vi "QBridge 0MQ focuser.vi"() -> (0 "error":errorcluster)   [LabVIEW 2018]
uses:
  <vilib>/addons/zeromq/zmq_socket.lvclass
  <vilib>/addons/zeromq/zmq_context.lvclass
  <vilib>/addons/zeromq/socket_type.ctl
  <vilib>/addons/zeromq/socket_options.ctl
  <vilib>/addons/zeromq/zeromq.lvlib
panel:
  out "focuserREP message":string
  out "Focuser160_REQ":string caption="Message to Focuser160"
  out "Focus Status":string
  in  "QueueBaseName":string="focusQueue"
  in  "stop":bool
  # "QBRIDGE ZeroMQ Focuser"
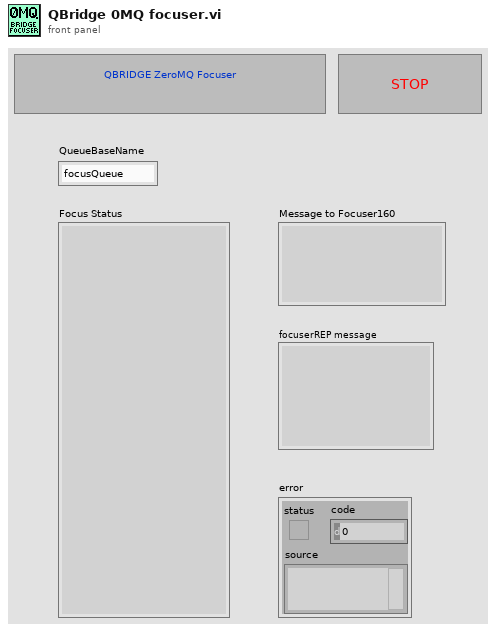
[diagram p1: front panel]
types:
  T1 = typedef "zeromq.lvlib/socket_options.ctl" = enum8{"NONE", "ZMQ_HWM", "<2>", "ZMQ_SWAP", "ZMQ_AFFINITY", "ZMQ_ROUTING_ID", "ZMQ_SUBSCRIBE", "ZMQ_UNSUBSCRIBE", "ZMQ_RATE", "ZMQ_RECOVERY_IVL", "ZMQ_MCAST_LOOP", "ZMQ_SNDBUF", "ZMQ_RCVBUF", "ZMQ_RCVMORE", "ZMQ_FD", "ZMQ_EVENTS", "ZMQ_TYPE", "ZMQ_LINGER", "ZMQ_RECONNECT_IVL", "ZMQ_BACKLOG", "ZMQ_RECOVERY_IVL_MSEC", "ZMQ_RECONNECT_IVL_MAX", "ZMQ_MAXMSGSIZE", "ZMQ_SNDHWM", "ZMQ_RCVHWM", "ZMQ_MULTICAST_HOPS", "<26>", "ZMQ_RCVTIMEO", "ZMQ_SNDTIMEO", "<29>", "<30>", "ZMQ_IPV4ONLY", "ZMQ_LAST_ENDPOINT", "ZMQ_ROUTER_MANDATORY", "ZMQ_TCP_KEEPALIVE", "ZMQ_TCP_KEEPALIVE_CNT", "ZMQ_TCP_KEEPALIVE_IDLE", "ZMQ_TCP_KEEPALIVE_INTVL", "ZMQ_TCP_ACCEPT_FILTER", "ZMQ_IMMEDIATE", "ZMQ_XPUB_VERBOSE", "ZMQ_ROUTER_RAW", "ZMQ_IPV6", "ZMQ_MECHANISM", "ZMQ_PLAIN_SERVER", "ZMQ_PLAIN_USERNAME", "ZMQ_PLAIN_PASSWORD", "ZMQ_CURVE_SERVER", "ZMQ_CURVE_PUBLICKEY", "ZMQ_CURVE_SECRETKEY", "ZMQ_CURVE_SERVERKEY", "ZMQ_PROBE_ROUTER", "ZMQ_REQ_CORRELATE", "ZMQ_REQ_RELAXED", "ZMQ_CONFLATE", "ZMQ_ZAP_DOMAIN", "ZMQ_ROUTER_HANDOVER", "ZMQ_TOS", "ZMQ_IPC_FILTER_PID", "ZMQ_IPC_FILTER_UID", "ZMQ_IPC_FILTER_GID", "ZMQ_CONNECT_ROUTING_ID", "ZMQ_GSSAPI_SERVER", "ZMQ_GSSAPI_PRINCIPAL", "ZMQ_GSSAPI_SERVICE_PRINCIPAL", "ZMQ_GSSAPI_PLAINTEXT", "ZMQ_HANDSHAKE_IVL", "<67>", "ZMQ_SOCKS_PROXY", "ZMQ_XPUB_NODROP", "ZMQ_BLOCKY", "ZMQ_XPUB_MANUAL", "ZMQ_XPUB_WELCOME_MSG", "ZMQ_STREAM_NOTIFY", "ZMQ_INVERT_MATCHING", "ZMQ_HEARTBEAT_IVL", "ZMQ_HEARTBEAT_TTL", "ZMQ_HEARTBEAT_TIMEOUT", "ZMQ_XPUB_VERBOSER", "ZMQ_CONNECT_TIMEOUT", "ZMQ_TCP_MAXRT", "ZMQ_THREAD_SAFE", "<82>", "<83>", "ZMQ_MULTICAST_MAXTPDU", "ZMQ_VMCI_BUFFER_SIZE", "ZMQ_VMCI_BUFFER_MIN_SIZE", "ZMQ_VMCI_BUFFER_MAX_SIZE", "ZMQ_VMCI_CONNECT_TIMEOUT", "ZMQ_USE_FD", "ZMQ_GSSAPI_PRINCIPAL_NAMETYPE", "ZMQ_GSSAPI_SERVICE_PRINCIPAL_NAMETYPE", "ZMQ_BINDTODEVICE", "ZMQ_ZAP_ENFORCE_DOMAIN", "ZMQ_LOOPBACK_FASTPATH", "ZMQ_METADATA", "ZMQ_MULTICAST_LOOP", "ZMQ_ROUTER_NOTIFY"}
  T2 = typedef "zeromq.lvlib/socket_type.ctl" = enum8{"ZMQ_PAIR", "ZMQ_PUB", "ZMQ_SUB", "ZMQ_REQ", "ZMQ_REP", "ZMQ_DEALER", "ZMQ_ROUTER", "ZMQ_PULL", "ZMQ_PUSH", "ZMQ_XPUB", "ZMQ_XSUB", "ZMQ_STREAM", "ZMQ_SERVER", "ZMQ_CLIENT", "ZMQ_RADIO", "ZMQ_DISH", "ZMQ_GATHER", "ZMQ_SCATTER", "ZMQ_DGRAM"}
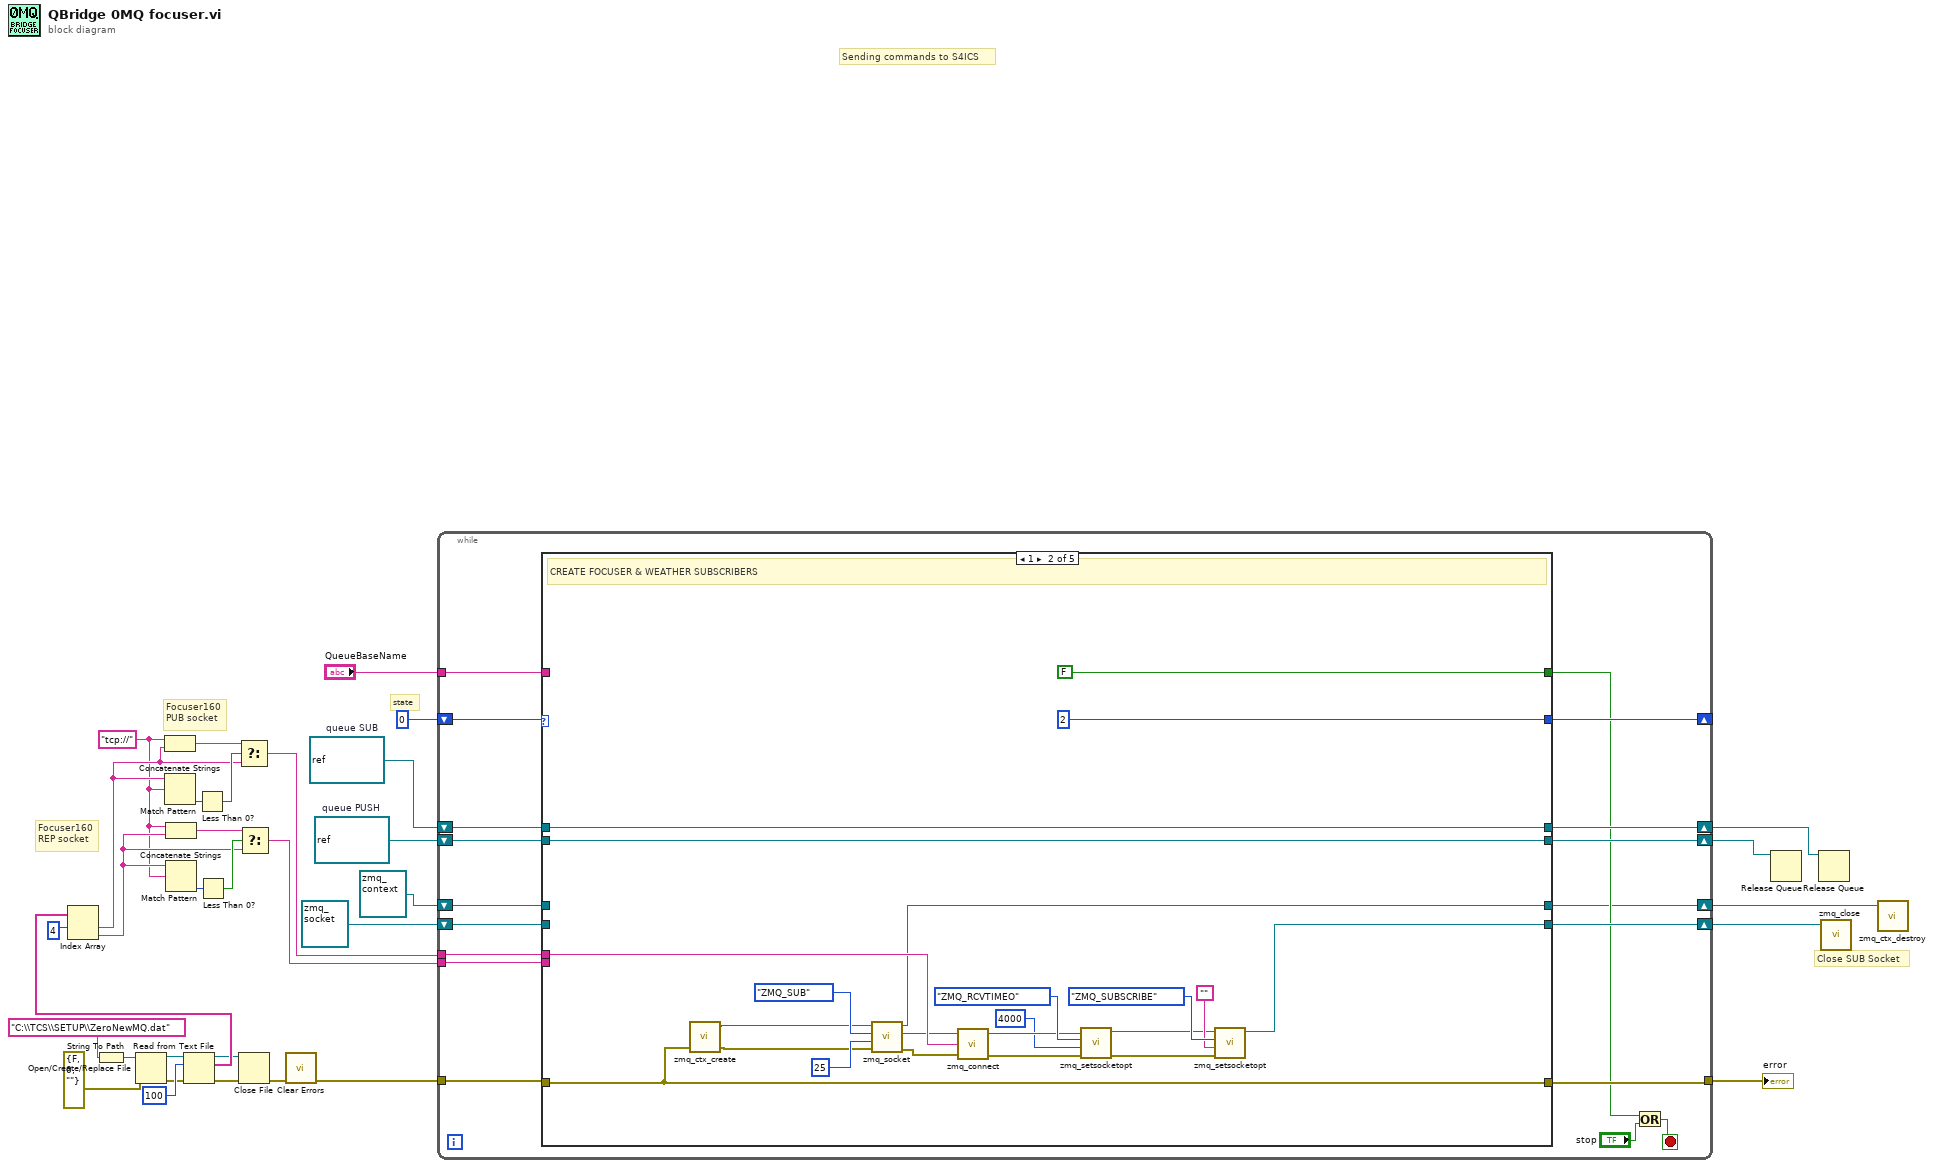
[diagram p0: block diagram]
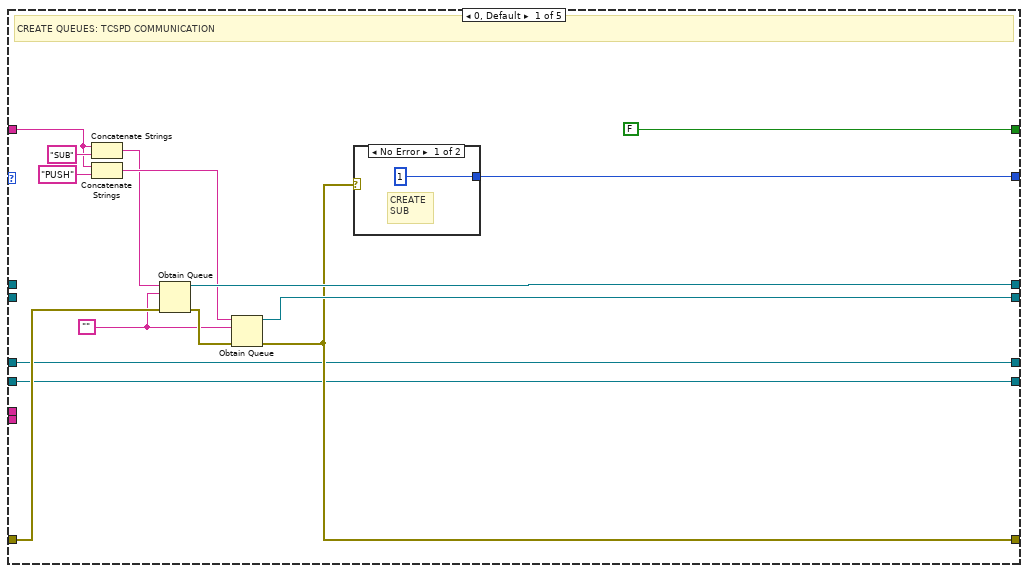
[diagram p2: hidden frame]
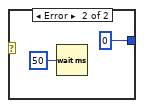
[diagram p3: hidden frame]
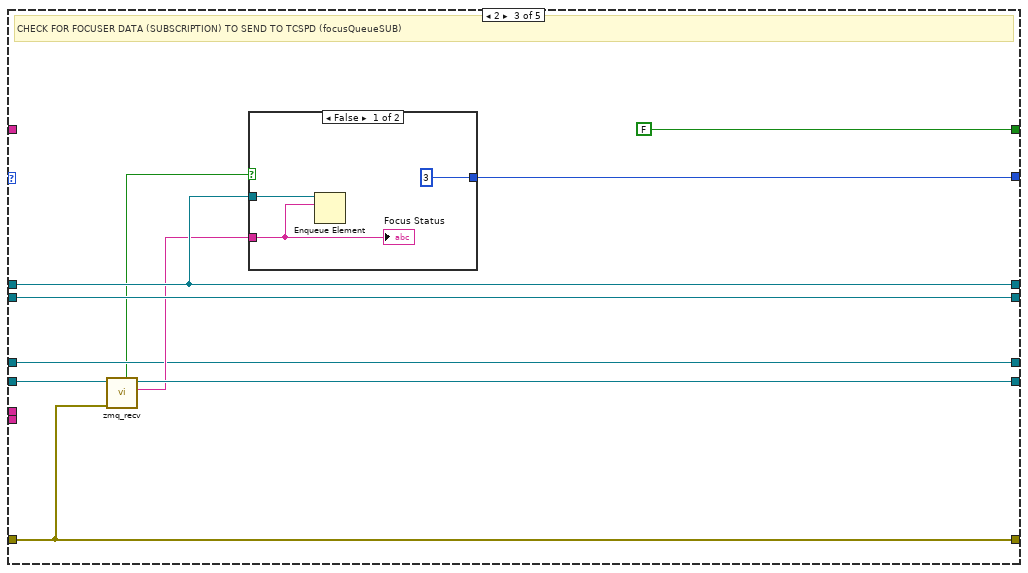
[diagram p4: hidden frame]
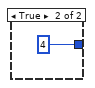
[diagram p5: hidden frame]
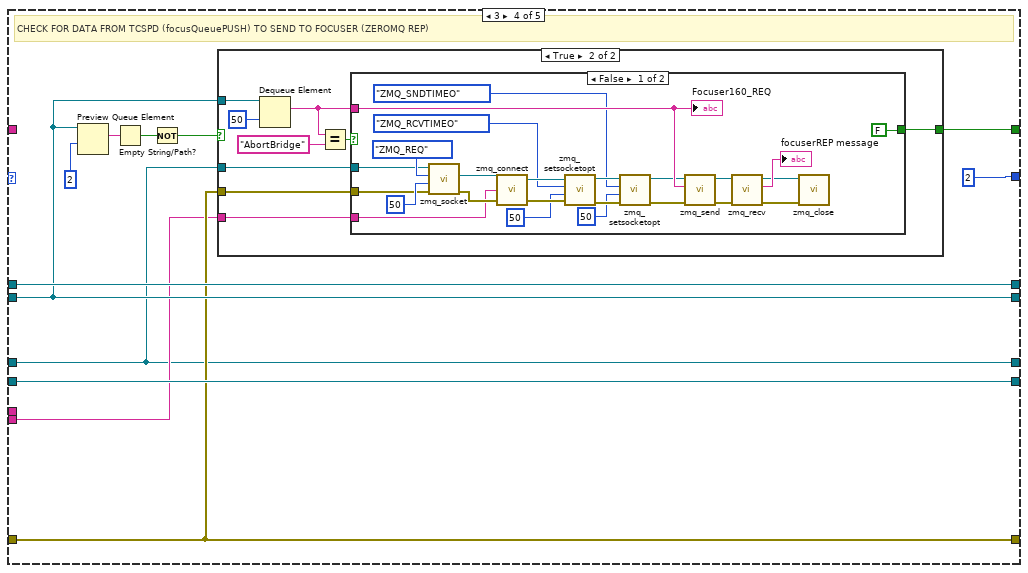
[diagram p6: hidden frame]
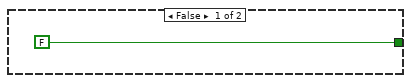
[diagram p7: hidden frame]
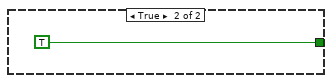
[diagram p8: hidden frame]
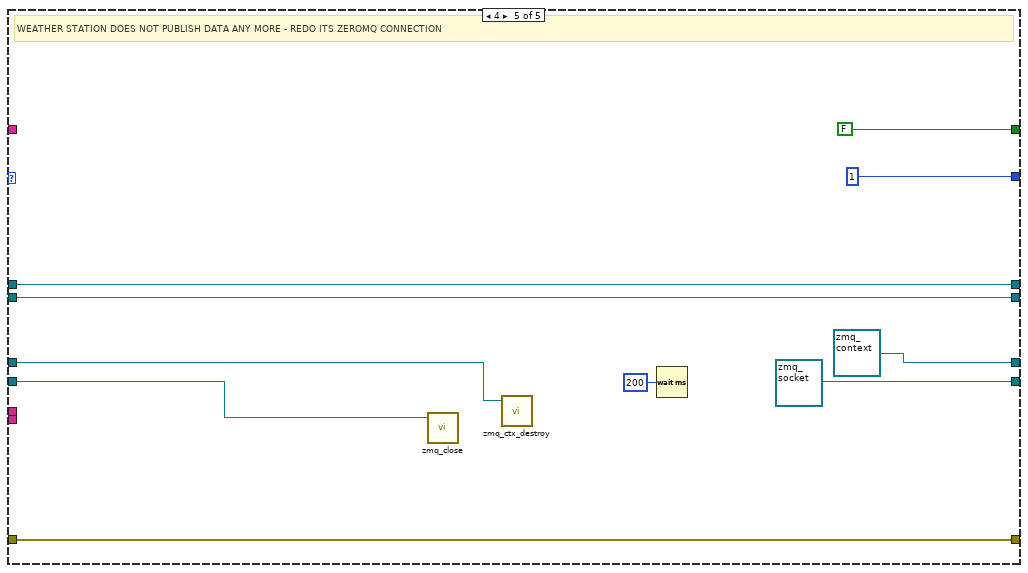
[diagram p9: hidden frame]
diagram:
  w4 = "tcp://"
  w32 = refnum<queue> refnum  # queue PUSH
  w31 = refnum<queue> refnum  # queue SUB
  # "Close SUB Socket"
  # "Focuser160\nREP socket"
  # "Focuser160\nPUB socket"
  # "state"
  # "Sending commands to S4ICS"
  n1 = String To Path(string="C:\\TCS\\SETUP\\ZeroNewMQ.dat") -> (path=w29:path)
  n2 = Open/Create/Replace File(file path (use dialog)=w29, error in=errorcluster {"status"=FALSE, "code"=0, "source"=""}) -> (refnum out=w27:refnum<file>, error out=w20:errorcluster)  [unwired: 4 in, 1 out]
  n3 = Read from Text File(file (use dialog)=w27, count=100, error in=w20) -> (refnum out=w23:refnum<file>, text=w25:string[], error out=w16:errorcluster)  [unwired: 1 in, 1 out]
  n4 = Index Array(array=w25, index #1=4 ("index")) -> (element #1=w6:string, element #2=w11:string)  [unwired: 1 in]
  n5 = Concatenate Strings(w4, w6) -> (w8:string)
  n6 = Match Pattern(string=w6, regular expression=w4) -> (offset past match=w7:i32)  [unwired: 1 in, 3 out]
  n7 = Concatenate Strings(w4, w11) -> (w13:string)
  n8 = Match Pattern(string=w11, regular expression=w4) -> (offset past match=w12:i32)  [unwired: 1 in, 3 out]
  n9 = Less Than 0?(x=w7) -> (x < 0?=w9:bool)
  n10 = Less Than 0?(x=w12) -> (x < 0?=w14:bool)
  n11 = Select(t=w8, s=w9, f=w6) -> (s? t:f=w5:string)
  n12 = Close File(refnum=w23, error in=w16) -> (error out=w17:errorcluster)  [unwired: 1 out]
  n13 = Select(t=w13, s=w14, f=w11) -> (s? t:f=w10:string)
  n14 = call <vilib>:"Clear Errors.vi"("error in (no error)"=w17) -> ("error out"=w3:errorcluster)  [unwired: 5 in, 1 out]
  n15 = while {
    shift-right: [w50] -> _
    shift-left: u16 0 -> [w52]
    shift-right: [w46] -> w19
    shift-left: w31 -> [w44]
    shift-right: [w45] -> w18
    shift-left: w32 -> [w43]
    tunnel: w3 -> [w51]
    tunnel: [w49] -> w33
    tunnel: "QueueBaseName" -> [w42]
    tunnel: w5 -> [w41]
    tunnel: w10 -> [w40]
    shift-right: [w38] -> w15
    shift-left: refnum<class "zmq_socket.lvclass"> refnum ("socket out") -> [w39]
    shift-right: [w35] -> w1
    shift-left: refnum<class "zmq_context.lvclass"> refnum ("context out") -> [w36]
    stop <- w47 stop-if-true
    n16 = case shown="1" w52 {
      tunnel: w51 -> [w64 w81 w97 w112 w161]
      tunnel: [w65 u16 2 w93 u16 2 u16 1] -> w50
      tunnel: [w62 w81 w97 w112 w161] -> w49
      tunnel: [w67 w91 w99 w118 w163] -> w46
      tunnel: [w66 w90 w102 w114 w162] -> w45
      tunnel: w44 -> [_ w91 w99 w118 w163]
      tunnel: w43 -> [_ w90 w102 w114 w162]
      tunnel: w42 -> [w56 _ _ _ _]
      tunnel: w41 -> [_ w88 _ _ _]
      tunnel: w40 -> [_ _ _ w109 _]
      tunnel: w39 -> [w55 _ w101 w113 w158]
      tunnel: [w55 w92 w100 w113 refnum<class "zmq_socket.lvclass"> refnum ("socket out")] -> w38
      tunnel: [FALSE FALSE FALSE w111 FALSE] -> w37
      tunnel: w36 -> [w53 _ w95 w107 w157]
      tunnel: [w53 w77 w95 w107 refnum<class "zmq_context.lvclass"> refnum ("context out")] -> w35
      frame 0, Default {
        w57 = ""
        # "CREATE QUEUES: TCSPD COMMUNICATION"
        n17 = Concatenate Strings(w56, "SUB" ("string")) -> (w58:string)
        n18 = Concatenate Strings(w56, "PUSH" ("string")) -> (w60:string)
        n19 = Obtain Queue(name (unnamed)=w58, element data type=w57, error in (no error)=w64) -> (queue out=w67:refnum<queue>, error out=w63:errorcluster)  [unwired: 2 in, 1 out]
        n20 = Obtain Queue(name (unnamed)=w60, element data type=w57, error in (no error)=w63) -> (queue out=w66:refnum<queue>, error out=w62:errorcluster)  [unwired: 2 in, 1 out]
        n21 = case shown="No Error" w62 {
          tunnel: [u16 1 u16 0] -> w65
          frame No Error {
            # "CREATE\nSUB"
          }
          frame Error {
            n22 = Wait (ms)(milliseconds to wait=u32 50) -> ()  [unwired: 1 out]
          }
        }
      }
      frame 1 {
        # "CREATE FOCUSER & WEATHER SUBSCRIBERS"
        n23 = call <vilib>:"zmq_ctx_create.vi"("error in"=w81) -> ("error out"=w78:errorcluster, "context out"=w79:refnum<class "zmq_context.lvclass">)  [unwired: 3 in]
        n24 = call <vilib>:"zmq_socket.vi"("error in"=w78, "linger (ms)"=25, "socket type"=socket_type."ZMQ_SUB", "context in"=w79) -> ("error out"=w86:errorcluster, "socket out"=w87:refnum<class "zmq_socket.lvclass">, "context out"=w77:refnum<class "zmq_context.lvclass">)  [unwired: 1 in]
        n25 = call <vilib>:"zmq_connect.vi"("error in"=w86, "endpoint"=w88, "socket in"=w87) -> ("error out"=w72:errorcluster, "socket out"=w75:refnum<class "zmq_socket.lvclass">)  [unwired: 1 in]
        n26 = call <vilib>:"zmq_setsocketopt.vi"("error in"=w72, "value"=u16 4000, "option"=socket_options."ZMQ_RCVTIMEO", "socket in"=w75) -> ("error out"=w73:errorcluster, "socket out"=w74:refnum<class "zmq_socket.lvclass">)  [unwired: 2 in]
        n27 = call <vilib>:"zmq_setsocketopt.vi"("error in"=w73, "value"="", "option"=socket_options."ZMQ_SUBSCRIBE", "socket in"=w74) -> ("socket out"=w92:refnum<class "zmq_socket.lvclass">)  [unwired: 2 in, 1 out]
      }
      frame 2 {
        # "CHECK FOR FOCUSER DATA (SUBSCRIPTION) TO SEND TO TCSPD (focusQueueSUB)"
        n28 = call <vilib>:"zmq_recv.vi"("error in"=w97, "socket in"=w101) -> ("data"=w96:string, "socket out"=w100:refnum<class "zmq_socket.lvclass">, "timeout?"=w94:bool)  [unwired: 3 in, 2 out]
        n29 = case shown="False" w94 {
          tunnel: w99 -> [w105 _]
          tunnel: w96 -> [w104 _]
          tunnel: [u16 3 u16 4] -> w93
          frame False {
            n30 = Enqueue Element(queue=w105, element=w104) -> ()  [unwired: 2 in, 3 out]
            "Focus Status" <- w104
          }
          frame True {
          }
        }
      }
      frame 3 {
        # "CHECK FOR DATA FROM TCSPD (focusQueuePUSH) TO SEND TO FOCUSER (ZEROMQ REP)"
        n31 = Preview Queue Element(queue=w114, timeout in ms (-1)=2) -> (element=w117:string)  [unwired: 1 in, 3 out]
        n32 = Empty String/Path?(string/path=w117) -> (empty?=w116:bool)
        n33 = Not(x=w116) -> (.not. x?=w115:bool)
        n34 = case shown="True" w115 {
          tunnel: w114 -> [_ w128]
          tunnel: w109 -> [_ w126]
          tunnel: w112 -> [_ w127]
          tunnel: [FALSE w122] -> w111
          tunnel: w107 -> [_ w120]
          frame False {
          }
          frame True {
            n35 = Dequeue Element(queue=w128, timeout in ms (-1)=50) -> (element=w124:string)  [unwired: 1 in, 3 out]
            n36 = Equal?(x=w124, y="AbortBridge") -> (x = y?=w123:bool)
            n37 = case shown="False" w123 {
              tunnel: w127 -> [w145 _]
              tunnel: w126 -> [w150 _]
              tunnel: w124 -> [w149 _]
              tunnel: [FALSE TRUE] -> w122
              tunnel: w120 -> [w129 _]
              frame False {
                n38 = call <vilib>:"zmq_socket.vi"("error in"=w145, "linger (ms)"=50, "socket type"=socket_type."ZMQ_REQ", "context in"=w129) -> ("error out"=w152:errorcluster, "socket out"=w151:refnum<class "zmq_socket.lvclass">)  [unwired: 1 in, 1 out]
                n39 = call <vilib>:"zmq_connect.vi"("error in"=w152, "endpoint"=w150, "socket in"=w151) -> ("error out"=w139:errorcluster, "socket out"=w138:refnum<class "zmq_socket.lvclass">)  [unwired: 1 in]
                n40 = call <vilib>:"zmq_setsocketopt.vi"("error in"=w139, "value"=50 ("linger (ms)"), "option"=socket_options."ZMQ_RCVTIMEO", "socket in"=w138) -> ("error out"=w136:errorcluster, "socket out"=w135:refnum<class "zmq_socket.lvclass">)  [unwired: 2 in]
                n41 = call <vilib>:"zmq_setsocketopt.vi"("error in"=w136, "value"=50 ("linger (ms)"), "option"=socket_options."ZMQ_SNDTIMEO", "socket in"=w135) -> ("error out"=w131:errorcluster, "socket out"=w130:refnum<class "zmq_socket.lvclass">)  [unwired: 2 in]
                n42 = call <vilib>:"zmq_send.vi"("error in"=w131, "data"=w149, "socket in"=w130) -> ("error out"=w144:errorcluster, "socket out"=w143:refnum<class "zmq_socket.lvclass">)  [unwired: 4 in]
                n43 = call <vilib>:"zmq_recv.vi"("error in"=w144, "socket in"=w143) -> ("error out"=w140:errorcluster, "data"=→"focuserREP message":string, "socket out"=w141:refnum<class "zmq_socket.lvclass">)  [unwired: 3 in, 2 out]
                n44 = call <vilib>:"zmq_close.vi"("error in"=w140, "socket"=w141) -> ()  [unwired: 3 in, 1 out]
                "Focuser160_REQ" <- w149
              }
              frame True {
              }
            }
          }
        }
      }
      frame 4 {
        # "WEATHER STATION DOES NOT PUBLISH DATA ANY MORE - REDO ITS ZEROMQ CONNECTION"
        n45 = call <vilib>:"zmq_close.vi"("socket"=w158) -> ()  [unwired: 4 in, 1 out]
        n46 = call <vilib>:"zmq_ctx_destroy.vi"("context in"=w157) -> ()  [unwired: 4 in, 1 out]
        n47 = Wait (ms)(milliseconds to wait=u32 200) -> ()  [unwired: 1 out]
      }
    }
    n48 = Or(x=w37, y="stop") -> (x .or. y?=w47:bool)
  }
  "error" <- w33
  n49 = Release Queue(queue=w18) -> ()  [unwired: 2 in, 3 out]
  n50 = Release Queue(queue=w19) -> ()  [unwired: 2 in, 3 out]
  n51 = call <vilib>:"zmq_close.vi"("socket"=w15) -> ()  [unwired: 4 in, 1 out]
  n52 = call <vilib>:"zmq_ctx_destroy.vi"("context in"=w1) -> ()  [unwired: 4 in, 1 out]
